vi "Measurement Logic.vi"() -> ()   [LabVIEW 2021, in "Efficiency Sweep_Class D Amplifier.lvlib"]
uses:
  Efficiency Sweep_Class D Amplifier.lvlib
  Measurement Results.ctl
  <vilib>/Analysis/NI_AALBase.lvlib
  <vilib>/MeasurementLink/MeasurementLink Measurement Server/Measure Call Context/Measure Call Context.lvclass
  <vilib>/Analysis/1siggen.llb/Ramp Pattern by Samples.vi
  Measurement Configuration.ctl
  shared/controls/single tone audio measurements.ctl
  shared/controls/audio controls.lvlib
  shared/controls/digital audio protocol/data justification.ctl
  shared/controls/digital audio protocol/endianness.ctl
  shared/controls/digital audio protocol/digital edge.ctl
  shared/controls/digital audio protocol/logic level.ctl
  shared/controls/weighting filter.ctl
  shared/controls/lowpass filter.ctl
  shared/controls/highpass filter.ctl
  shared/controls/sweep profile.ctl
  shared/controls/units - snr.ctl
  shared/controls/units - ratio.ctl
  shared/controls/digital output level units.ctl
  shared/controls/regulation target.ctl
  shared/controls/regulation target value units.ctl
panel:
  out "results":T1={"channel"="0", "frequency (Hz)"=1000.0000024177915, "amplitude (Vrms)"=-6.256665451281146, "amplitude (dBFS)"=78.42395339546047, "phase (deg)"=0.0, "SNR"=-71.07176133726693, "THD+N"=-71.98384642729017, "THD"=-0.25666545128114626, "dynamic range (dB)"=83.34902670182771, "gain"=102.93430172121762, "SFDR (dBc)"=0.0}
  out "Spectrum":cluster{"x0":dbl, "dx":dbl, "magnitude":dbl[]}(graph)
  out "Waveform Graph":waveform(dbl)(graph)
  out "measure call context out":refnum<class "Measure Call Context.lvclass">
  in  "measure call context in":refnum<class "Measure Call Context.lvclass">
  out "measurement results":T2={"channel name"="0", "frequency (Hz)"=[], "amplitude (Vrms)"=[], "amplitude (dBFS)"=[], "SNR"=[], "THD+N"=[], "THD"=[], "dynamic range (dB)"=[], "gain"=[], "SFDR (dBc)"=[], "output power (W)"=[], "wfm - t0"=0.0, "wfm - dt"=1.9531249997269942e-05, "wfm - data"=array[12800 elements], "fft - f0"=0.0, "fft - df"=4.000000000559116, "fft - data"=array[6400 elements]}
  in  "measurement configuration":T3={"digital channel list"="7821\\PCMo 8", "frame clock rate"=48000.0, "number of channels"=2, "channel length"=32, "bit depth"=24, "data justification"=enum."Left Justified", "endianness"=enum."MSB First", "bit clock edge sync"=enum."Rising", "frame sync edge for channel 0"=enum."Rising", "channel 0 offset"=1, "master clock channel list"="7821\\PCMo 0", "master clock rate"=12288000.0, "enable dither"=TRUE, "logic level"=enum."3.3 V", "output level"=-10.0, "output level units"=enum."dBFS", "output range (pk-pk)"=15.0, "load impedance"=4.0, "signal phase"=0.0, "acq sampling rate"=51200.0, "min measurement cycles"=20, "min measurement time (s)"=0.1, "min settling cycles"=0, "min settling time (s)"=0.005, "acq channel"="PXI1Slot4/ai0", "band start"=20.0, "band stop"=20000.0, "weighting filter"=enum."Linear", "highpass filter"=enum."DC", "lowpass filter"=enum."No filter", "sweep start frequency (Hz)"=20.0, "sweep stop frequency (Hz)"=20000.0, "number of steps"=10, "sweep profile"=enum."Logarithmic", "SNR units"=enum."dB", "THD+N units"=enum."dB", "THD units"=enum."dB", "gain units"=enum."dB", "enable regulation"=FALSE, "regulation target"=enum."THD+N Ratio", "regulation target value"=10.0, "regulation target value units"=enum."%", "regulation start level"=-1.0, "regulation stop level"=-10.0, "regulation number of steps"=2} {"min measurement cycles" format="%0.2f"; "channel 0 offset" format="%#_6p"; "output range (pk-pk)" format="%0.2f"; "signal phase" format="%0.2f"; "frame clock rate" format="%#_6pHz"}
  out "error out":errorcluster
  in  "error in":errorcluster
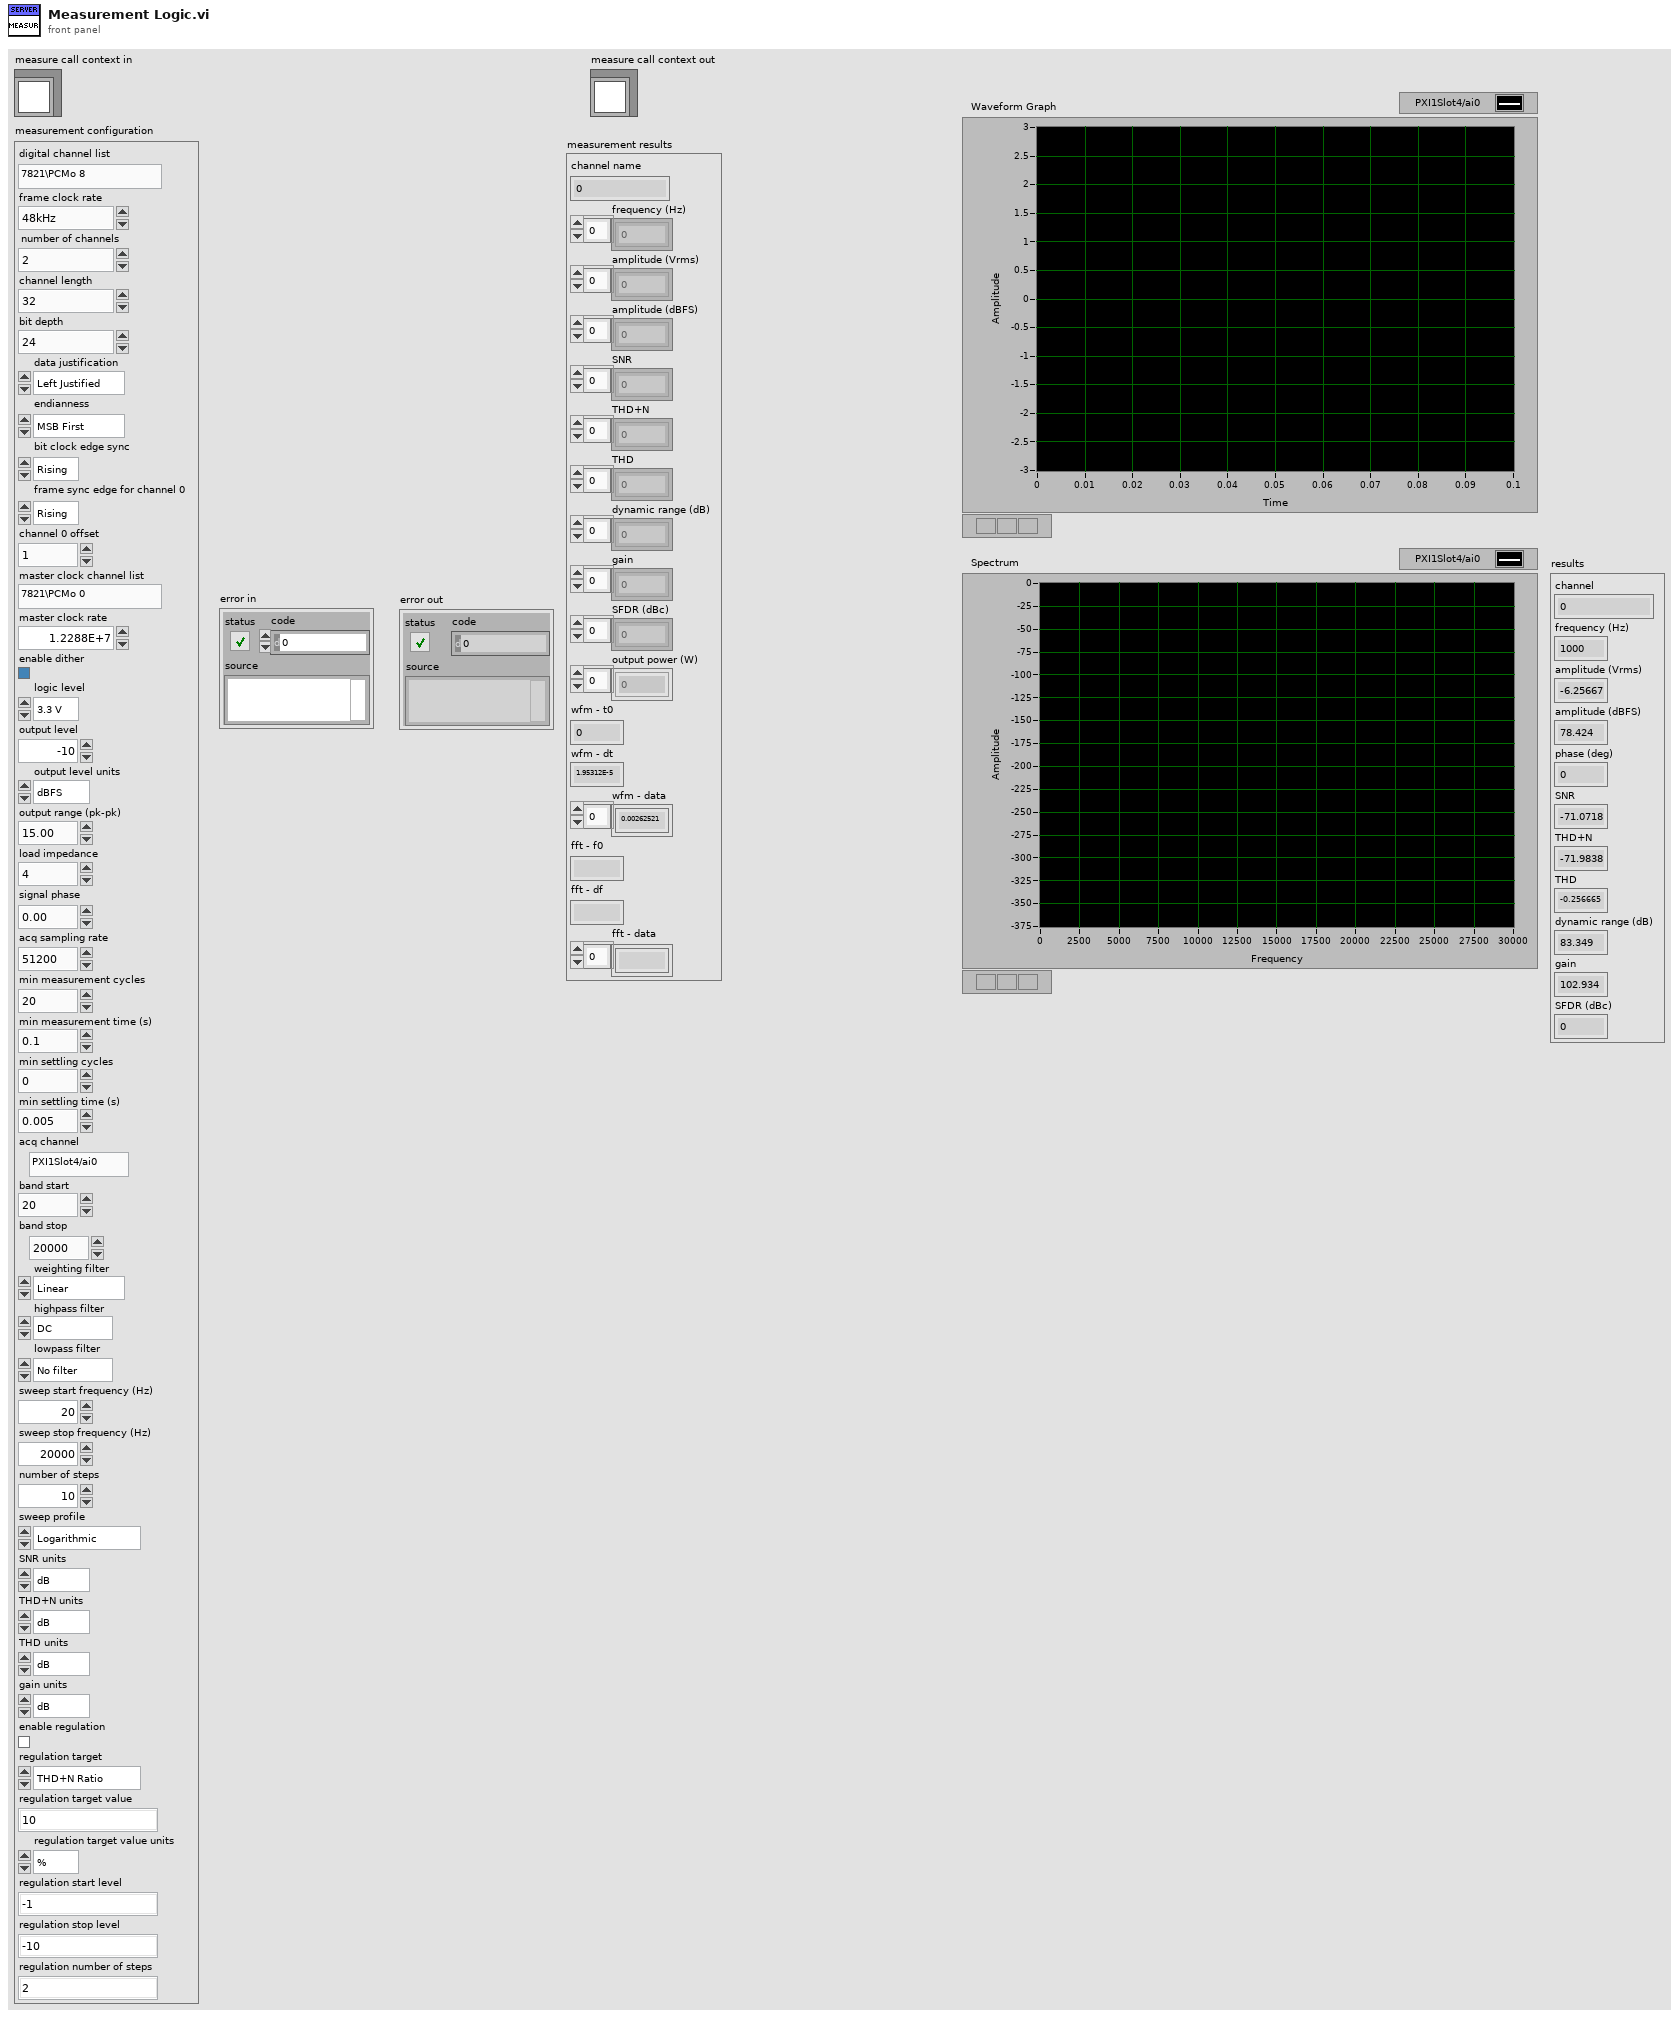
[diagram p1: front panel]
types:
  T1 = typedef "audio controls.lvlib/single tone audio measurements.ctl" = cluster{"channel":string, "frequency (Hz)":dbl, "amplitude (Vrms)":dbl, "amplitude (dBFS)":dbl, "phase (deg)":dbl, "SNR":dbl, "THD+N":dbl, "THD":dbl, "dynamic range (dB)":dbl, "gain":dbl, "SFDR (dBc)":dbl}
  T2 = typedef "Efficiency Sweep_Class D Amplifier.lvlib/Measurement Results.ctl" = cluster{"channel name":string, "frequency (Hz)":dbl[], "amplitude (Vrms)":dbl[], "amplitude (dBFS)":dbl[], "SNR":dbl[], "THD+N":dbl[], "THD":dbl[], "dynamic range (dB)":dbl[], "gain":dbl[], "SFDR (dBc)":dbl[], "output power (W)":dbl[], "wfm - t0":dbl, "wfm - dt":dbl, "wfm - data":dbl[], "fft - f0":dbl, "fft - df":dbl, "fft - data":dbl[]}
  T3 = typedef "Efficiency Sweep_Class D Amplifier.lvlib/Measurement Configuration.ctl" = cluster{"digital channel list":string, "frame clock rate":dbl, "number of channels":u32, "channel length":u32, "bit depth":u32, "data justification":T4, "endianness":T5, "bit clock edge sync":T6, "frame sync edge for channel 0":T6, "channel 0 offset":u32, "master clock channel list":string, "master clock rate":dbl, "enable dither":bool, "logic level":T7, "output level":dbl, "output level units":T8, "output range (pk-pk)":dbl, "load impedance":dbl, "signal phase":dbl, "acq sampling rate":dbl, "min measurement cycles":u32, "min measurement time (s)":dbl, "min settling cycles":u32, "min settling time (s)":dbl, "acq channel":string, "band start":dbl, "band stop":dbl, "weighting filter":T9, "highpass filter":T10, "lowpass filter":T11, "sweep start frequency (Hz)":dbl, "sweep stop frequency (Hz)":dbl, "number of steps":u32, "sweep profile":T12, "SNR units":T13, "THD+N units":T14, "THD units":T14, "gain units":T14, "enable regulation":bool, "regulation target":T15, "regulation target value":dbl, "regulation target value units":T16, "regulation start level":dbl, "regulation stop level":dbl, "regulation number of steps":u32}
  T4 = typedef "data justification.ctl" = enum32{"Left Justified", "Right Justified"}
  T5 = typedef "endianness.ctl" = enum32{"MSB First", "LSB First"}
  T6 = typedef "digital edge.ctl" = enum32{"Rising", "Falling"}
  T7 = typedef "logic level.ctl" = enum32{"3.3 V", "1.8 V", "1.2 V"}
  T8 = typedef "audio controls.lvlib/digital output level units.ctl" = enum32{"% FS", "dBFS"}
  T9 = typedef "weighting filter.ctl" = enum32{"Linear", "A-weighting", "B-weighting", "C-weighting"}
  T10 = typedef "highpass filter.ctl" = enum32{"DC", "AC"}
  T11 = typedef "lowpass filter.ctl" = enum32{"No filter", "AES17 20kHz", "AES17 40kHz"}
  T12 = typedef "audio controls.lvlib/sweep profile.ctl" = enum32{"Linear", "Logarithmic"}
  T13 = typedef "audio controls.lvlib/units - snr.ctl" = enum32{"dB", "x/y"}
  T14 = typedef "audio controls.lvlib/units - ratio.ctl" = enum32{"dB", "%", "x/y"}
  T15 = typedef "regulation target.ctl" = enum32{"THD+N Ratio", "Output Power"}
  T16 = typedef "regulation target value units.ctl" = enum32{"%", "W"}
  T17 = typedef "regulation settings.ctl" = cluster{"enable regulation":bool, "regulation target":T15, "regulation target value":dbl, "regulation target value units":T16, "regulation start level":dbl, "regulation stop level":dbl, "regulation number of steps":u32}
  T18 = typedef "single tone measurement settings (HW).ctl" = cluster{"digital channel list":string, "frame clock rate":dbl, "number of channels":u32, "channel length":u32, "bit depth":u32, "data justification":T4, "endianness":T5, "bit clock edge sync":T6, "frame sync edge for channel 0":T6, "channel 0 offset":u32, "master clock channel list":string, "master clock rate":dbl, "enable dither":bool, "logic level":T7, "signal frequency":dbl, "output level":dbl, "output level units":T8, "output range (pk-pk)":dbl, "load impedance":dbl, "signal phase":dbl, "acq sampling rate":dbl, "min measurement cycles":u32, "min measurement time (s)":dbl, "min settling cycles":u32, "min settling time (s)":dbl, "acq channel":string, "band start":dbl, "band stop":dbl, "weighting filter":T9, "highpass filter":T10, "lowpass filter":T11, "SNR units":T13, "THD+N units":T14, "THD units":T14, "gain units":T14}
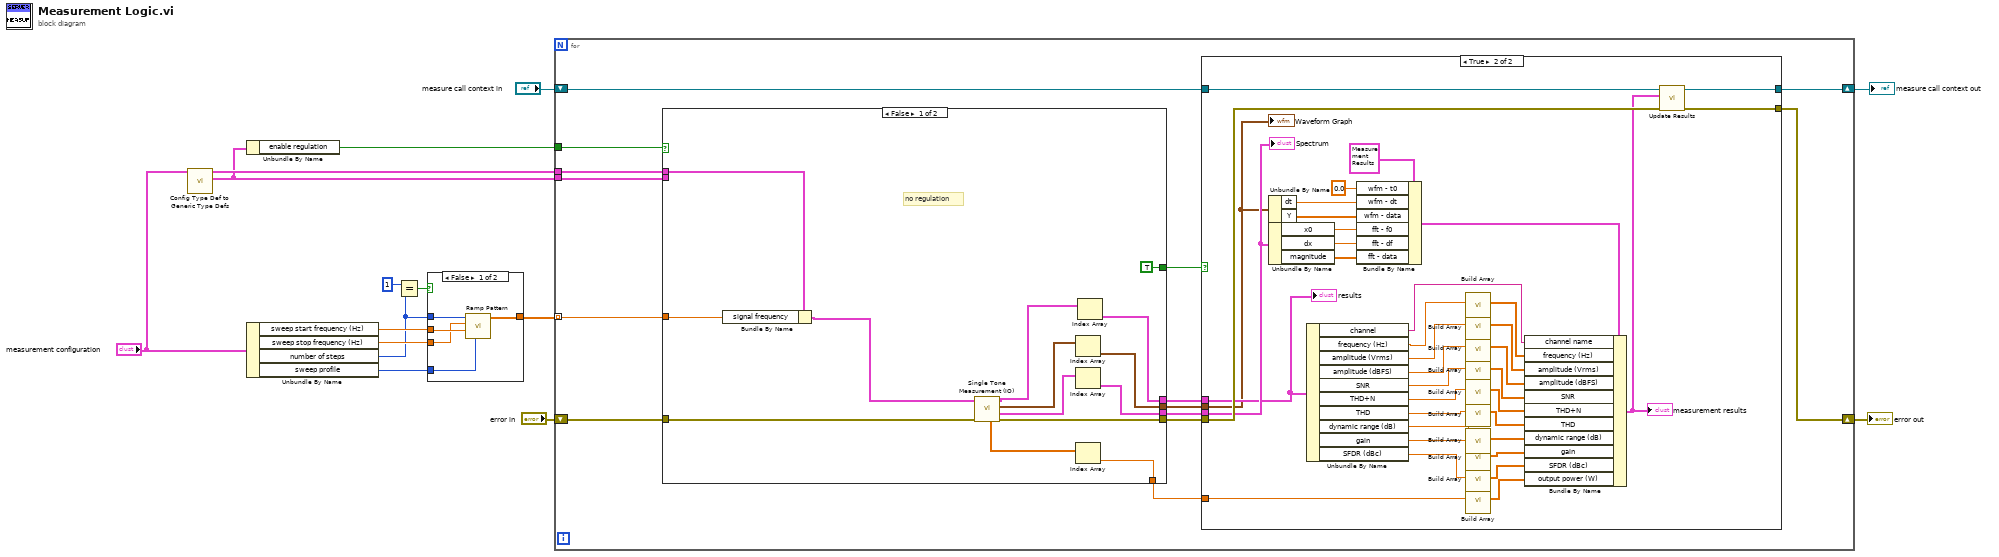
[diagram p0: block diagram]
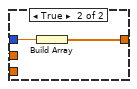
[diagram p2: hidden frame]
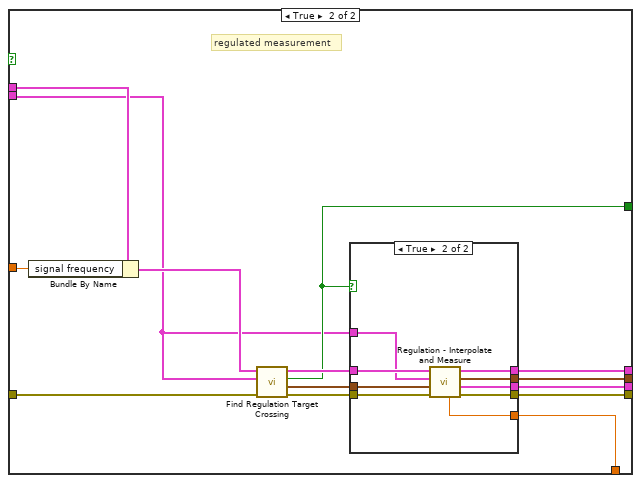
[diagram p4: hidden frame]
diagram:
  n1 = call "Config Type Def to Generic Type Defs.vi"("measurement configuration"="measurement configuration") -> ("regulation settings"=w1:T17, "single tone settings"=w2:T18)  [unwired: 9 in]
  n2 = Unbundle By Name(w1) -> ("enable regulation"=w4:bool)
  n3 = Unbundle By Name("measurement configuration") -> ("sweep start frequency (Hz)"=w14:dbl, "sweep stop frequency (Hz)"=w13:dbl, "number of steps"=w7:u32, "sweep profile"=w15:T12)
  n4 = Equal?(x=u32 1, y=w7) -> (x = y?=w8:bool)
  n5 = case shown="False" w8 {
    tunnel: w15 -> [w20 _]
    tunnel: w14 -> [w19 w22]
    tunnel: w13 -> [w18 _]
    tunnel: w7 -> [w17 _]
    tunnel: [w16 w21] -> w12
    frame False {
      n6 = call-poly <vilib>:"Ramp Pattern.vi"("type"=w20, "start"=w19, "end"=w18, "samples"=w17) -> ("Ramp Pattern"=w16:dbl[])  [unwired: 6 in, 1 out]
    }
    frame True {
      n7 = Build Array(w22) -> (w21:dbl[])
    }
  }
  n8 = for {
    tunnel: w12 -> [w28] mode=indexing
    shift-right: [w33] -> w10
    shift-left: "error in" -> [w36]
    shift-right: [w34] -> w9
    shift-left: "measure call context in" -> [w32]
    tunnel: w4 -> [w27]
    tunnel: w2 -> [w24]
    tunnel: w1 -> [w23]
    n9 = case shown="False" w27 {
      tunnel: w36 -> [w89 w103]
      tunnel: [w88 w101] -> w35
      tunnel: [w80 w96] -> w31
      tunnel: [w78 w95] -> w30
      tunnel: [w76 w98] -> w29
      tunnel: w28 -> [w85 w93]
      tunnel: [w81 w97] -> w26
      tunnel: [TRUE ("crossing found?") w94] -> w25
      tunnel: w24 -> [w86 w92]
      tunnel: w23 -> [_ w90]
      frame False {
        # "no regulation"
        n10 = Bundle By Name(cluster=w86, "signal frequency"=w85) -> (w84:T18)
        n11 = call "Single Tone Measurement (IO).vi"("error in (no error)"=w89, "measurement configuration"=w84) -> ("error out"=w88:errorcluster, "spectra"=w82:cluster{"x0":dbl, "dx":dbl, "magnitude":dbl[]}[], "waveforms"=w83:waveform(dbl)[], "results"=w77:T1[], "output power"=w79:dbl[])  [unwired: 4 in, 1 out]
        n12 = Index Array(array=w83) -> (element=w81:waveform(dbl))  [unwired: 1 in]
        n13 = Index Array(array=w82) -> (element=w80:cluster{"x0":dbl, "dx":dbl, "magnitude":dbl[]})  [unwired: 1 in]
        n14 = Index Array(array=w79) -> (element=w78:dbl)  [unwired: 1 in]
        n15 = Index Array(array=w77) -> (element=w76:T1)  [unwired: 1 in]
      }
      frame True {
        # "regulated measurement"
        n16 = Bundle By Name(cluster=w92, "signal frequency"=w93) -> (w91:T18)
        n17 = call "Find Regulation Target Crossing.vi"("error in (no error)"=w103, "regaultion settings"=w90, "measurement configuration"=w91) -> ("error out"=w102:errorcluster, "search results"=w99:cluster{"level":dbl, "value":dbl}[], "crossing found?"=w94:bool, "measurement configuration out"=w100:T18)  [unwired: 5 in]
        n18 = case shown="True" w94 {
          tunnel: w102 -> [w104 w112]
          tunnel: [w104 w110] -> w101
          tunnel: w100 -> [_ w113]
          tunnel: w99 -> [_ w111]
          tunnel: [_ w109] -> w98
          tunnel: [_ w108] -> w97
          tunnel: [_ w107] -> w96
          tunnel: [_ w106] -> w95
          tunnel: w90 -> [_ w105]
          frame False {
            # "could not regulate to value"
          }
          frame True {
            n19 = call "Regulation - Interpolate and Measure.vi"("error in (no error)"=w112, "search results"=w111, "regulation settings"=w105, "measurement configuration"=w113) -> ("error out"=w110:errorcluster, "spectrum"=w107:cluster{"x0":dbl, "dx":dbl, "magnitude":dbl[]}, "time domain"=w108:waveform(dbl), "results"=w109:T1, "output power"=w106:dbl)  [unwired: 2 in, 1 out]
          }
        }
      }
    }
    n20 = case shown="True" w25 {
      tunnel: w35 -> [w37 w75]
      tunnel: [w38 w74] -> w34
      tunnel: [w37 w73] -> w33
      tunnel: w32 -> [w38 w72]
      tunnel: w31 -> [_ w71]
      tunnel: w30 -> [_ w70]
      tunnel: w29 -> [_ w69]
      tunnel: w26 -> [_ w41]
      frame False {
        # "could not regulate, do not add measurement"
      }
      frame True {
        n21 = Unbundle By Name(w41) -> ("dt"=w40:dbl, "Y"=w39:dbl[])
        n22 = Unbundle By Name(w71) -> ("x0"=w67:dbl, "dx"=w66:dbl, "magnitude"=w65:dbl[])
        n23 = Unbundle By Name(w69) -> ("channel"=w42:string, "frequency (Hz)"=w43:dbl, "amplitude (Vrms)"=w44:dbl, "amplitude (dBFS)"=w45:dbl, "SNR"=w46:dbl, "THD+N"=w47:dbl, "THD"=w48:dbl, "dynamic range (dB)"=w49:dbl, "gain"=w50:dbl, "SFDR (dBc)"=w51:dbl)
        n24 = Bundle By Name(cluster=T2 {"channel name"="", "frequency (Hz)"=[], "amplitude (Vrms)"=[], "amplitude (dBFS)"=[], "SNR"=[], "THD+N"=[], "THD"=[], "dynamic range (dB)"=[], "gain"=[], "SFDR (dBc)"=[], "output power (W)"=[], "wfm - t0"=0.0, "wfm - dt"=0.0, "wfm - data"=[], "fft - f0"=0.0, "fft - df"=0.0, "fft - data"=[]} ("Measurement Results"), "wfm - t0"=0.0, "wfm - dt"=w40, "wfm - data"=w39, "fft - f0"=w67, "fft - df"=w66, "fft - data"=w65) -> (w63:T2)
        n25 = call "Build Array.vi"("value"=w43) -> ("Array"=w62:dbl[])  [unwired: 10 in]
        n26 = call "Build Array.vi"("value"=w44) -> ("Array"=w61:dbl[])  [unwired: 10 in]
        n27 = call "Build Array.vi"("value"=w45) -> ("Array"=w60:dbl[])  [unwired: 10 in]
        n28 = call "Build Array.vi"("value"=w46) -> ("Array"=w58:dbl[])  [unwired: 10 in]
        n29 = call "Build Array.vi"("value"=w47) -> ("Array"=w57:dbl[])  [unwired: 10 in]
        n30 = call "Build Array.vi"("value"=w48) -> ("Array"=w56:dbl[])  [unwired: 10 in]
        n31 = call "Build Array.vi"("value"=w49) -> ("Array"=w55:dbl[])  [unwired: 10 in]
        n32 = call "Build Array.vi"("value"=w50) -> ("Array"=w54:dbl[])  [unwired: 10 in]
        n33 = call "Build Array.vi"("value"=w51) -> ("Array"=w53:dbl[])  [unwired: 10 in]
        n34 = call "Build Array.vi"("value"=w70) -> ("Array"=w52:dbl[])  [unwired: 10 in]
        n35 = Bundle By Name(cluster=w63, "channel name"=w42, "frequency (Hz)"=w62, "amplitude (Vrms)"=w61, "amplitude (dBFS)"=w60, "SNR"=w58, "THD+N"=w57, "THD"=w56, "dynamic range (dB)"=w55, "gain"=w54, "SFDR (dBc)"=w53, "output power (W)"=w52) -> (w59:T2)
        "measurement results" <- w59
        n36 = call <vilib>:"Update Results.vi"("error in"=w75, "measurement results"=w59, "measure call context in"=w72) -> ("error out"=w73:errorcluster, "measure call context out"=w74:refnum<class "Measure Call Context.lvclass">)  [unwired: 7 in]
        "Waveform Graph" <- w41
        "Spectrum" <- w71
        "results" <- w69
      }
    }
  }
  "error out" <- w10
  "measure call context out" <- w9
